vi "SpectraData2.vi"() -> ()   [LabVIEW 2015]
panel:
  out "Waveform Graph":dbl[][](graph)
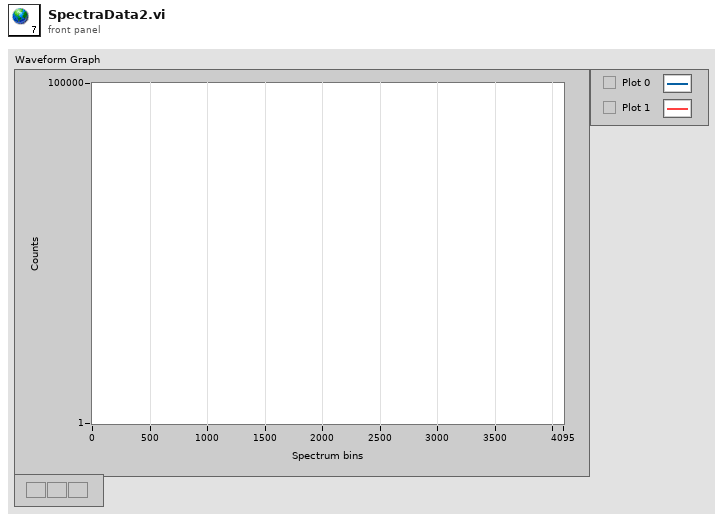
[diagram p1: front panel]
diagram:
